vi "ASCII Streaming Instrument.vi"() -> ()   [LabVIEW 2019]
uses:
  <vilib>/numeric/Random Number (Range) DBL.vi
  <vilib>/Instr/_visa.llb/VISA Configure Serial Port (Instr).vi
panel:
  out "read buffer":string
  out "error out":errorcluster
  in  "stop":bool
  in  "VISA resource name":refnum<visa-resource-name>
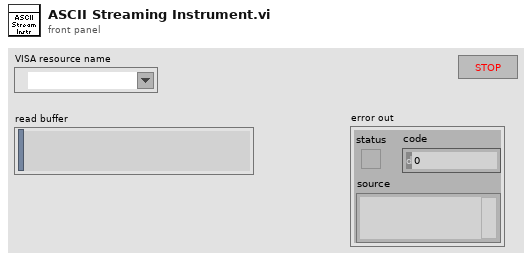
[diagram p1: front panel]
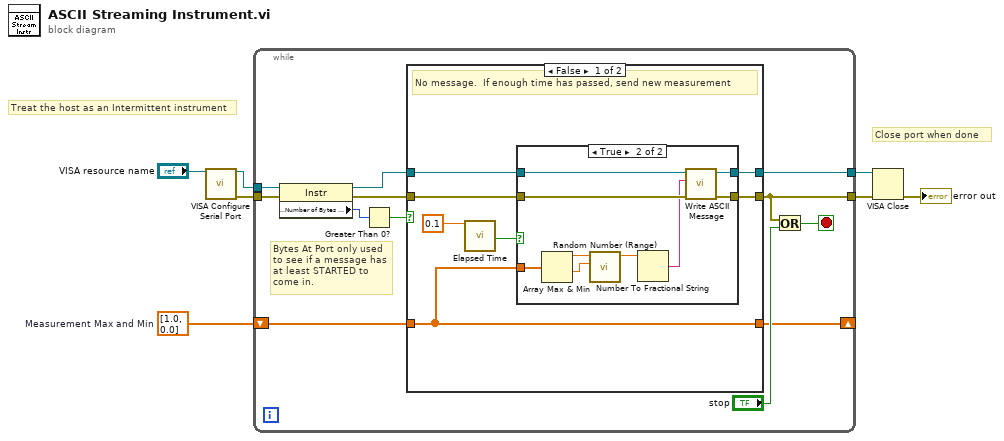
[diagram p0: block diagram]
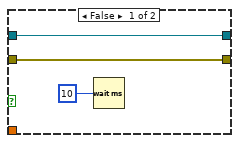
[diagram p2: hidden frame]
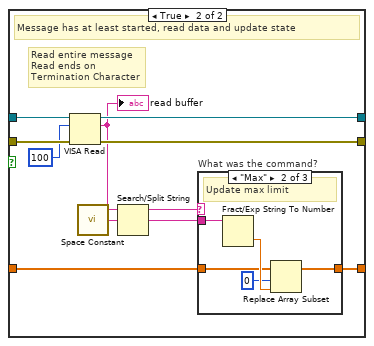
[diagram p3: hidden frame]
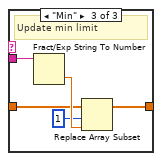
[diagram p5: hidden frame]
diagram:
  w2 = dbl[] [1.0, 0.0]  # Measurement Max and Min
  # "Treat the host as an Intermittent instrument"
  # "Close port when done"
  n1 = call-poly "VISA Configure Serial Port"("VISA resource name"="VISA resource name") -> ("VISA resource name out"=w1:refnum<visa-resource-name>, "error out"=w5:errorcluster)  [unwired: 13 in]
  n2 = while {
    tunnel: w5 -> [w19]
    tunnel: w1 -> [w16]
    tunnel: [w12] -> w3
    tunnel: [w17] -> w7
    shift-right: [w8] -> _
    shift-left: w2 -> [w9]
    stop <- w11 stop-if-true
    # "Bytes At Port only used\nto see if a message has\nat least STARTED to\ncome in."
    n3 = property class="Instr"(reference=w16, error in=w19) -> (reference out=w13:refnum<visa-resource-name>, error out=w18:errorcluster, "Serial Settings:Number of Bytes at Serial Port"=w15:u32)
    n4 = Greater Than 0?(x=w15) -> (x > 0?=w14:bool)
    n5 = case shown="False" w14 {
      tunnel: w18 -> [w26 w49]
      tunnel: w13 -> [w23 w47]
      tunnel: [w20 w45] -> w12
      tunnel: [w25 w48] -> w17
      tunnel: w9 -> [w21 w40]
      tunnel: [w21 w39] -> w8
      frame False {
        # "No message.  If enough time has passed, send new measurement"
        n6 = call "Elapsed Time"("Time Target (s)"=0.1) -> ("Time has Elapsed"=w22:bool)  [unwired: 11 in, 7 out]
        n7 = case shown="True" w22 {
          tunnel: w23 -> [w28 w32]
          tunnel: w26 -> [w29 w38]
          tunnel: w21 -> [_ w36]
          tunnel: [w28 w31] -> w20
          tunnel: [w29 w37] -> w25
          frame False {
            n8 = Wait (ms)(milliseconds to wait=u32 10) -> ()  [unwired: 1 out]
          }
          frame True {
            n9 = Array Max & Min(array=w36) -> (max value=w35:dbl, min value=w34:dbl)  [unwired: 2 out]
            n10 = call-poly <vilib>:"Random Number (Range).vi"("lower bound (0)"=w34, "upper bound (100)"=w35) -> ("number"=w33:dbl)  [unwired: 9 in]
            n11 = Number To Fractional String(number=w33) -> (F-format string=w30:string)  [unwired: 3 in]
            n12 = call "Write ASCII Message.vi"("error in"=w38, "Message"=w30, "VISA resource in"=w32) -> ("error out"=w37:errorcluster, "VISA resource out"=w31:refnum<visa-resource-name>)  [unwired: 7 in]
          }
        }
      }
      frame True {
        # "Read entire message\nRead ends on\nTermination Character"
        # "Message has at least started, read data and update state"
        n13 = VISA Read(VISA resource name=w47, byte count=u32 100, error in (no error)=w49) -> (VISA resource name out=w45:refnum<visa-resource-name>, read buffer=w44:string, error out=w48:errorcluster)  [unwired: 1 out]
        "read buffer" <- w44
        n14 = call <vilib>:"Space Constant.vi"() -> ("String"=w43:string)
        n15 = Search/Split String(string=w44, search string/char (-)=w43) -> (substring before match=w42:string, match + rest of string=w41:string)  [unwired: 1 in, 1 out]
        n16 = case "What was the command?" shown="\"Max\"" w42 {
          tunnel: w41 -> [_ w54 w59]
          tunnel: w40 -> [w50 w53 w58]
          tunnel: [w50 w51 w56] -> w39
          frame Default {
            # "Unknown command"
          }
          frame "Max" {
            # "Update max limit"
            n17 = Fract/Exp String To Number(string=w54) -> (number=w55:dbl)  [unwired: 3 in, 1 out]
            n18 = Replace Array Subset(array=w53, new element=w55, index=0) -> (w51:dbl[])
          }
          frame "Min" {
            # "Update min limit"
            n19 = Fract/Exp String To Number(string=w59) -> (number=w60:dbl)  [unwired: 3 in, 1 out]
            n20 = Replace Array Subset(array=w58, new element=w60, index=1) -> (w56:dbl[])
          }
        }
      }
    }
    n21 = Or(x=w17, y="stop") -> (x .or. y?=w11:bool)
  }
  n22 = VISA Close(VISA resource name=w3, error in (no error)=w7) -> (error out=→"error out":errorcluster)
